vi "Read AONames.vi"(8 "error in (no error)":errorcluster, 11 "AO in":T1) -> (0 "error out":errorcluster, 2 "AONames":string[][](array[string]), 3 "AO out":T1)   [LabVIEW 2019, in "Inputs.lvlib"]
uses:
  Inputs.lvlib
  Ctl/AO.ctl
  Ctl/Parameter State.ctl
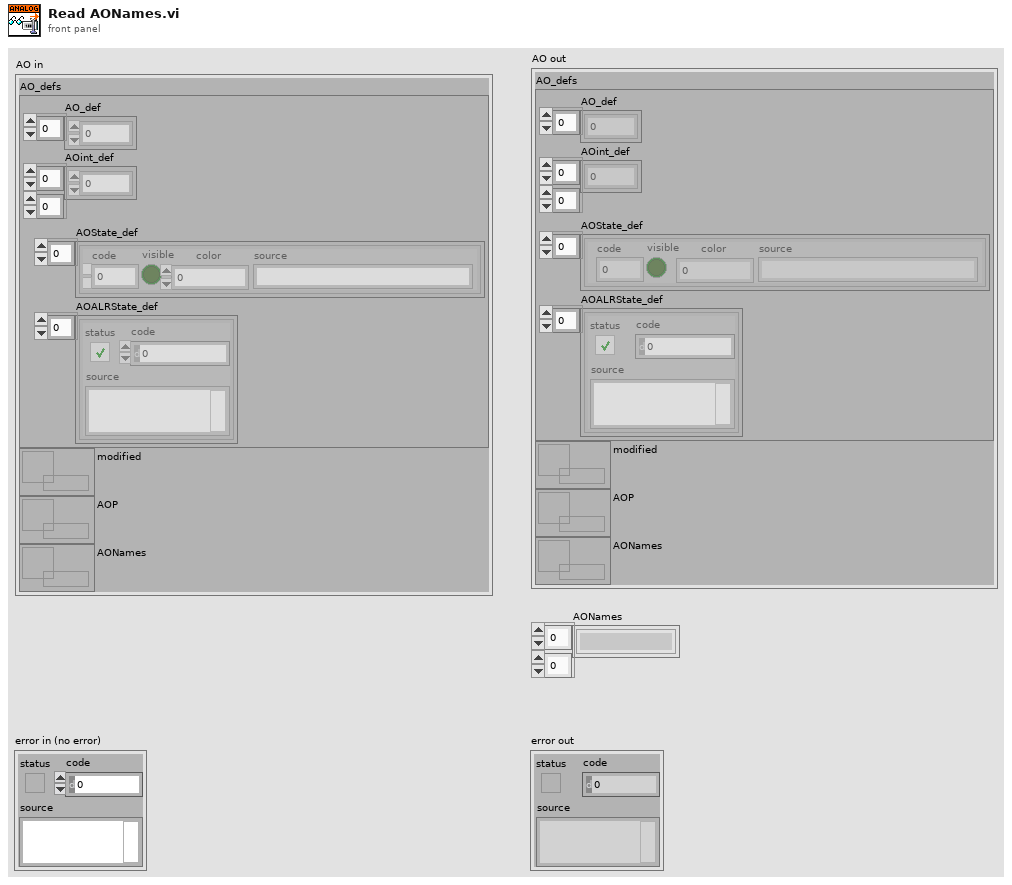
[diagram p1: front panel]
types:
  T1 = typedef "Inputs.lvlib/AO.ctl" = cluster{"AO_defs":cluster{"AO_def":dbl[], "AOint_def":u16[][], "AOState_def":T2[], "AOALRState_def":errorcluster[]}, "modified":refnum<data-value>, "AOP":refnum<data-value>, "AONames":refnum<data-value>}
  T2 = typedef "Inputs.lvlib/Parameter State.ctl" = cluster{"code":i32, "visible":bool, "color":u32, "source":string}
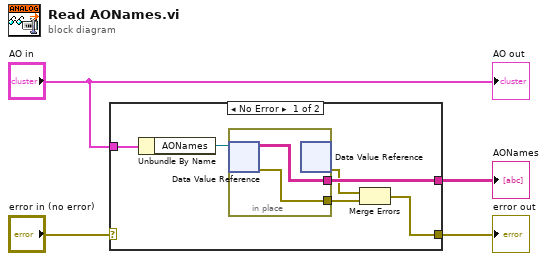
[diagram p0: block diagram]
diagram:
  n1 = case shown="No Error" "error in (no error)" {
    selector: "error in (no error)" -> [_ w13]
    tunnel: [w6 w13] -> w1
    tunnel: "AO in" -> [w5 _]
    tunnel: [w9 _] -> w2
    frame No Error {
      n2 = Unbundle By Name(w5) -> ("AONames"=w10:refnum<data-value>)
      n3 = in-place {
        in-place-border: [w12] -> w8
        in-place-border: [w11] -> w9
        n4 = in-place-dvr #1(w10) -> (w11:string[][], w12:errorcluster)
        n5 = in-place-dvr #1() -> (w7:errorcluster)  [unwired: 1 in, 1 out]
      }
      n6 = Merge Errors(w7, w8) -> (w6:errorcluster)
    }
    frame Error {
    }
  }
  "error out" <- w1
  "AONames" <- w2
  "AO out" <- "AO in"
